vi "scanning_FSM_main_AZ_ALT.vi"(4 "Time (ms)":u32, 6 "OK Button":bool, 7 "AZH":u16[](array[numeric]), 8 "ALT":u16[](array[numeric]), 9 "VISA resource name":refnum<visa-resource-name>) -> ()   [LabVIEW 2013]
uses:
  <vilib>/Instr/_visa.llb/VISA Configure Serial Port (Instr).vi
  <userlib>/Octoplus_LIDAR/GlobalNameAngles.vi
panel:
  out "ConcatenateAlt_Azh":string
  out "Current AZH":string
  out "return count 2":u16
  out "String sent AZH":string
  out "reverse azh":u16[](array[numeric])
  out "String sent ALT":string
  out "return count":u16
  out "Current ALT":string
  out "reverse alt":u16[](array[numeric])
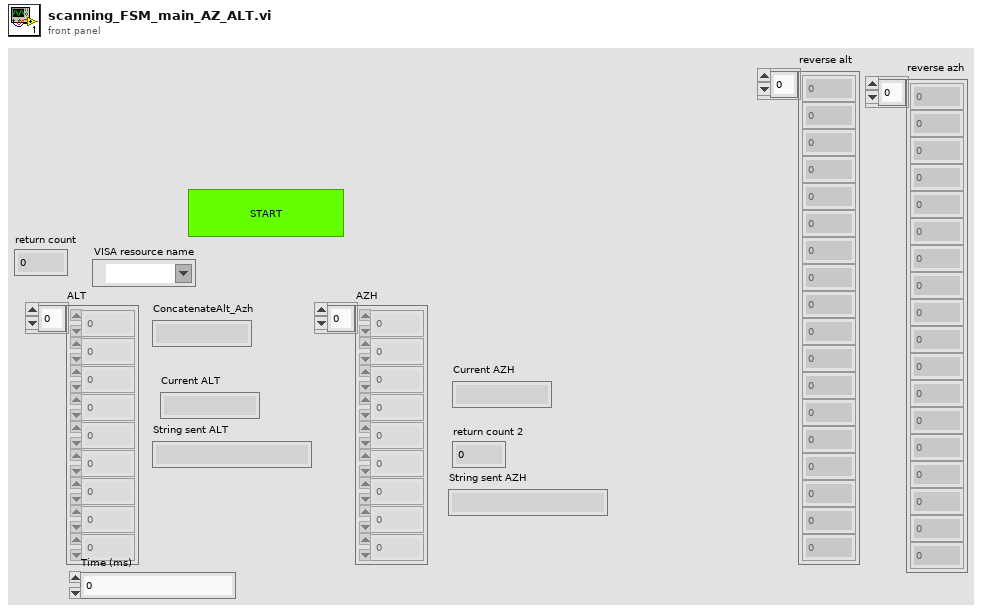
[diagram p1: front panel]
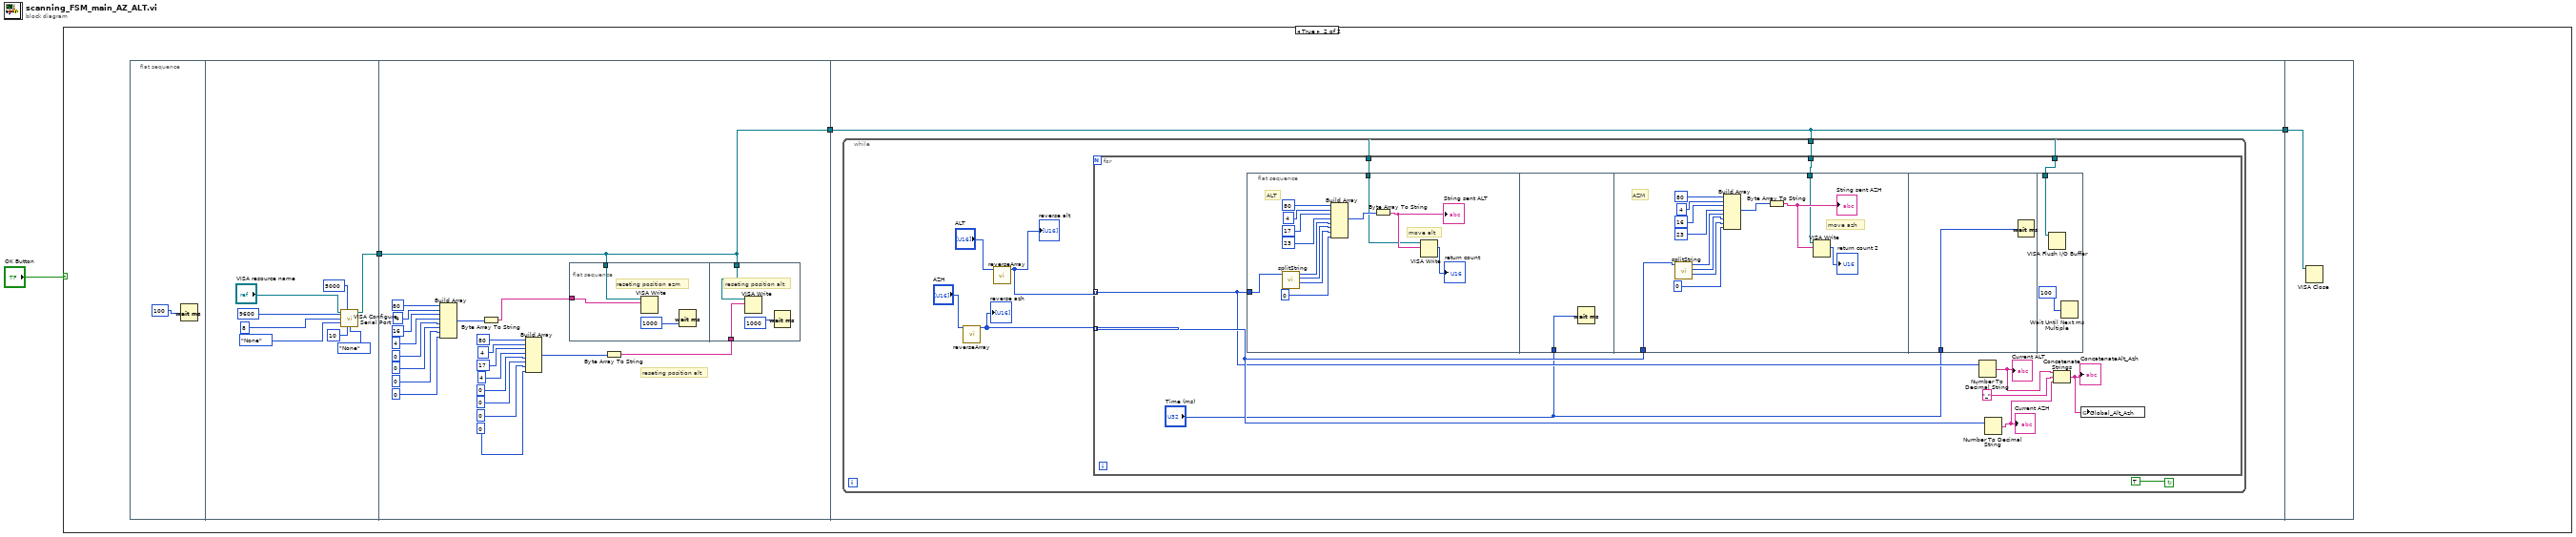
[diagram p0: block diagram]
diagram:
  n1 = case shown="True" "OK Button" {
    frame False {
    }
    frame True {
      n2 = flat-sequence {
        tunnel: [w7] -> w4
        tunnel: w4 -> [w14]
        tunnel: [w14] -> w3
        tunnel: w3 -> [w41]
        tunnel: [w41] -> w2
        tunnel: w2 -> [w88]
        frame #0 {
          n3 = Wait (ms)(milliseconds to wait=100) -> ()  [unwired: 1 out]
        }
        frame #1 {
          n4 = call-poly "VISA Configure Serial Port"("VISA resource name"="VISA resource name", "timeout (10sec)"=5000, "baud rate (9600)"=u32 9600, "data bits (8)"=u16 8, "parity (0:none)"=enum16{"None", "Odd", "Even", "Mark", "Space"}."None", "stop bits (10: 1 bit)"=10, "flow control (0:none)"=enum16{"", "None"}."None") -> ("VISA resource name out"=w7:refnum<visa-resource-name>)  [unwired: 7 in, 1 out]
        }
        frame #2 {
          # "reseting position alt"
          n5 = Build Array(u8 80, u8 4, u8 16, u8 4, u8 0, u8 0, u8 0, u8 0) -> (w34:u8[])
          n6 = Byte Array To String(unsigned byte array=w34) -> (string=w25:string)
          n7 = Build Array(u8 80, u8 4, u8 17, u8 4, u8 0, u8 0, u8 0, u8 0) -> (w24:u8[])
          n8 = flat-sequence {
            tunnel: w25 -> [w36]
            tunnel: w14 -> [w37]
            tunnel: w15 -> [w39]
            tunnel: w14 -> [w40]
            frame #0 {
              # "reseting position azm"
              n9 = VISA Write(VISA resource name=w37, write buffer=w36) -> ()  [unwired: 1 in, 3 out]
              n10 = Wait (ms)(milliseconds to wait=1000) -> ()  [unwired: 1 out]
            }
            frame #1 {
              # "reseting position alt"
              n11 = VISA Write(VISA resource name=w40, write buffer=w39) -> ()  [unwired: 1 in, 3 out]
              n12 = Wait (ms)(milliseconds to wait=1000) -> ()  [unwired: 1 out]
            }
          }
          n13 = Byte Array To String(unsigned byte array=w24) -> (string=w15:string)
        }
        frame #3 {
          n14 = while {
            tunnel: w41 -> [w47]
            stop <- TRUE continue-if-true
            n15 = call <userlib>:"reverseArray.vi"("angles: put 0 degree always as init angle"="AZH") -> ("Array out"=w44:u16[])  [unwired: 10 in]
            "reverse azh" <- w44
            n16 = call <userlib>:"reverseArray.vi"("angles: put 0 degree always as init angle"="ALT") -> ("Array out"=w43:u16[])  [unwired: 10 in]
            "reverse alt" <- w43
            n17 = for {
              tunnel: w43 -> [w53] mode=indexing
              tunnel: w44 -> [w54] mode=indexing
              tunnel: w47 -> [w57]
              tunnel: w47 -> [w56]
              tunnel: w47 -> [w55]
              n18 = flat-sequence {
                tunnel: w53 -> [w59]
                tunnel: w57 -> [w58]
                tunnel: "Time (ms)" -> [w71]
                tunnel: w54 -> [w74]
                tunnel: w56 -> [w72]
                tunnel: "Time (ms)" -> [w85]
                tunnel: w55 -> [w87]
                frame #0 {
                  # "ALT"
                  # "move alt"
                  n19 = call <userlib>:"splitString.vi"("Numeric"=w59) -> ("hex 3"=w62:u8, "hex 1"=w63:u8, "hex 0"=w64:u8)  [unwired: 8 in]
                  n20 = Build Array(u8 80, u8 4, u8 17, u8 23, w64, w63, w62, u8 0) -> (w70:u8[])
                  n21 = Byte Array To String(unsigned byte array=w70) -> (string=w60:string)
                  "String sent ALT" <- w60
                  n22 = VISA Write(VISA resource name=w58, write buffer=w60) -> (return count=→"return count":u32)  [unwired: 1 in, 2 out]
                }
                frame #1 {
                  n23 = Wait (ms)(milliseconds to wait=w71) -> ()  [unwired: 1 out]
                }
                frame #2 {
                  # "AZM"
                  # "move azh"
                  n24 = call <userlib>:"splitString.vi"("Numeric"=w74) -> ("hex 3"=w76:u8, "hex 1"=w77:u8, "hex 0"=w78:u8)  [unwired: 8 in]
                  n25 = Build Array(u8 80, u8 4, u8 16, u8 23, w78, w77, w76, u8 0) -> (w84:u8[])
                  n26 = Byte Array To String(unsigned byte array=w84) -> (string=w73:string)
                  "String sent AZH" <- w73
                  n27 = VISA Write(VISA resource name=w72, write buffer=w73) -> (return count=→"return count 2":u32)  [unwired: 1 in, 2 out]
                }
                frame #3 {
                  n28 = Wait (ms)(milliseconds to wait=w85) -> ()  [unwired: 1 out]
                }
                frame #4 {
                  n29 = VISA Flush I/O Buffer(VISA resource name=w87) -> ()  [unwired: 2 in, 2 out]
                  n30 = Wait Until Next ms Multiple(millisecond multiple=100) -> ()  [unwired: 1 out]
                }
              }
              n31 = Number To Decimal String(number=w53) -> (decimal integer string=w52:string)  [unwired: 1 in]
              "Current ALT" <- w52
              n32 = Number To Decimal String(number=w54) -> (decimal integer string=w51:string)  [unwired: 1 in]
              "Current AZH" <- w51
              n33 = Concatenate Strings(w52, "_", w51) -> (w48:string)
              "ConcatenateAlt_Azh" <- w48
              n34 = global write "GlobalNameAngles.vi" "Global_Alt_Azh"(w48) -> ()
            }
          }
        }
        frame #4 {
          n35 = VISA Close(VISA resource name=w88) -> ()  [unwired: 1 in, 1 out]
        }
      }
    }
  }
